vi "Periodic Tasks.vi"(8 "error in":errorcluster) -> ()   [LabVIEW 2017]
doc: "This VI runs in parallel to other tasks. It can contain as many user-defined periodic loops as you need. These can carry out PID or other sorts of timed response."
uses:
  <vilib>/Rock Robotics/WPI/Utilities/WPI_GetSetVariantRefNum.vi
  Robot Global Data.vi
  <vilib>/Rock Robotics/Network Tables/NT Write Numeric Array.vi
  <vilib>/Rock Robotics/Network Tables/NT Write Number.vi
  <vilib>/Rock Robotics/Network Tables/NT Write Boolean.vi
panel:
  out "ElevEnc":dbl
  out "LeftEncoder":dbl
  out "RightEncoder":dbl
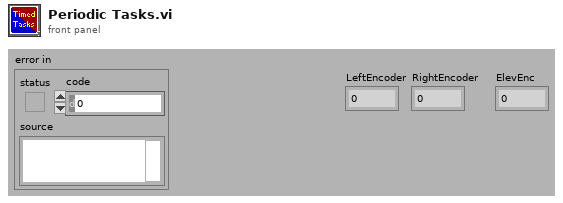
[diagram p1: front panel]
types:
  T1 = typedef "WPI_CompressorDevRef.ctl" = cluster{"DevStatus":errorcluster, "Pneumatics Control Module":u8}
  T2 = cluster{"Yaw":dbl, "Roll":dbl, "Pitch":dbl, "Heading":dbl, "Fused Heading":dbl}
  T3 = typedef "WPI_JoystickDevRef.ctl" = cluster{"Device":T4}
  T4 = typedef "WPI_JoystickDeviceEnum.ctl" = enum16{"USB 0", "USB 1", "USB 2", "USB 3", "USB 4", "USB 5"}
  T5 = typedef "WPI_DriverStationRobotMode2.ctl" = enum16{"Autonomous Disabled", "Autonomous Enabled", "Teleop Disabled", "Teleop Enabled", "Disconnected", "Finish", "Test Disabled", "Test Enabled", "Emergency Stopped"}
  T6 = cluster{"Buttons[0]":bool, "Buttons[1]":bool, "Buttons[2]":bool, "Buttons[3]":bool, "Buttons[4]":bool, "Buttons[5]":bool, "Buttons[6]":bool, "Buttons[7]":bool, "Buttons[8]":bool, "Buttons[9]":bool, "Buttons[10]":bool, "Buttons[11]":bool}
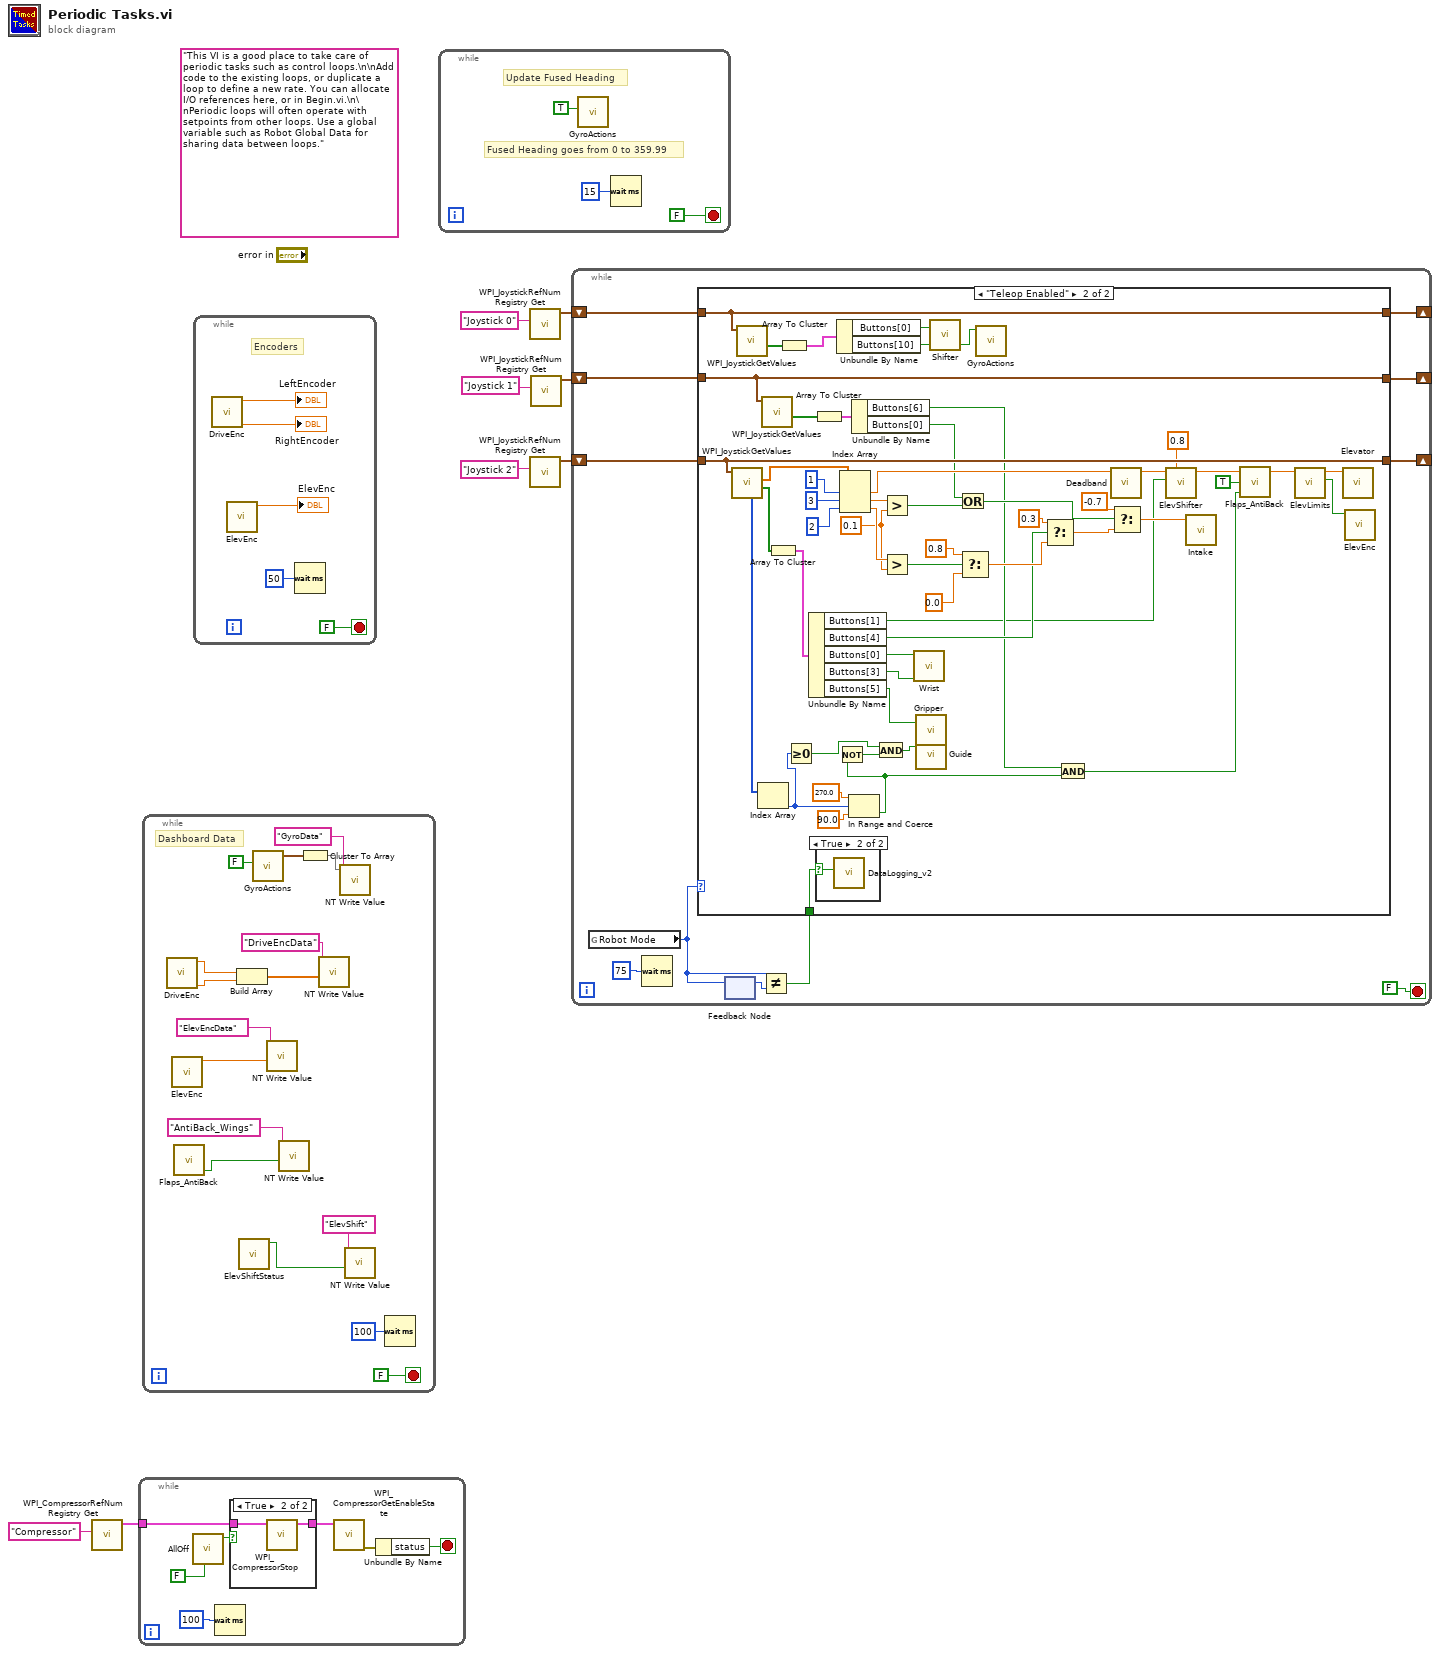
[diagram p0: block diagram]
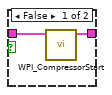
[diagram p4: hidden frame]
diagram:
  (unwired) "This VI is a good place to take care of periodic tasks such as control loops.\n\nAdd code to the existing loops, or duplicate a loop to define a new rate. You can allocate I/O references here, or in Begin.vi.\n\nPeriodic loops will often operate with setpoints from other loops. Use a global variable such as Robot Global Data for sharing data between loops."
  n1 = call <vilib>:"WPI_CompressorRefNum Registry Get.vi"("refnum name"="Compressor") -> ("CompressorDevRef"=w7:T1)  [unwired: 9 in, 1 out]
  n2 = while {
    tunnel: w7 -> [w13]
    stop <- w14 stop-if-true
    n3 = call "AllOff.vi"("Update?"=FALSE) -> ("Compressor"=w10:bool)  [unwired: 8 in, 2 out]
    n4 = Wait (ms)(milliseconds to wait=u32 100) -> ()  [unwired: 1 out]
    n5 = case shown="True" w10 {
      tunnel: w13 -> [w17 w19]
      tunnel: [w16 w18] -> w12
      frame False {
        n6 = call <vilib>:"WPI_CompressorStart.vi"("CompressorDevRef"=w17) -> ("CompressorDevRef"=w16:T1)  [unwired: 9 in, 1 out]
      }
      frame True {
        n7 = call <vilib>:"WPI_CompressorStop.vi"("CompressorDevRef"=w19) -> ("CompressorDevRef"=w18:T1)  [unwired: 9 in, 1 out]
      }
    }
    n8 = call <vilib>:"WPI_CompressorGetEnableState.vi"("CompressorDevRef"=w12) -> ("error out"=w11:errorcluster)  [unwired: 1 in, 9 out]
    n9 = Unbundle By Name(w11) -> ("status"=w14:bool)
  }
  n10 = while {
    stop <- FALSE stop-if-true
    # "Dashboard Data"
    n11 = call "DriveEnc.vi"() -> ("RightEncder"=w27:dbl, "LeftEncoder"=w28:dbl)  [unwired: 10 in]
    n12 = call "ElevEnc.vi"() -> ("ElevEnc"=w25:dbl)  [unwired: 11 in]
    n13 = call "Flaps_AntiBack.vi"() -> ("State"=w22:bool)  [unwired: 4 in, 1 out]
    n14 = Build Array(w28, w27) -> (w26:dbl[])
    n15 = call "ElevShiftStatus.vi"() -> ("ElevShiftStatusOut"=w20:bool)  [unwired: 11 in]
    n16 = call "GyroActions.vi"("Update?"=FALSE) -> ("YRPHfH"=w31:T2)  [unwired: 9 in, 1 out]
    n17 = call-poly <vilib>:"NT Write Value.vi"("Numeric"=w25, "Name"="ElevEncData") -> ()  [unwired: 9 in, 1 out]
    n18 = call-poly <vilib>:"NT Write Value.vi"("Boolean"=w22, "Name"="AntiBack_Wings") -> ()  [unwired: 9 in, 1 out]
    n19 = Cluster To Array(cluster=w31) -> (array=w35:dbl[])
    n20 = call-poly <vilib>:"NT Write Value.vi"("Numeric Array"=w26, "Name"="DriveEncData") -> ()  [unwired: 9 in, 1 out]
    n21 = call-poly <vilib>:"NT Write Value.vi"("Numeric Array"=w35, "Name"="GyroData") -> ()  [unwired: 9 in, 1 out]
    n22 = call-poly <vilib>:"NT Write Value.vi"("Boolean"=w20, "Name"="ElevShift") -> ()  [unwired: 9 in, 1 out]
    n23 = Wait (ms)(milliseconds to wait=u32 100) -> ()  [unwired: 1 out]
  }
  n24 = while {
    stop <- FALSE stop-if-true
    # "Encoders"
    n25 = call "DriveEnc.vi"() -> ("RightEncder"=→"RightEncoder":dbl, "LeftEncoder"=→"LeftEncoder":dbl)  [unwired: 10 in]
    n26 = call "ElevEnc.vi"() -> ("ElevEnc"=→"ElevEnc":dbl)  [unwired: 11 in]
    n27 = Wait (ms)(milliseconds to wait=u32 50) -> ()  [unwired: 1 out]
  }
  n28 = while {
    stop <- FALSE stop-if-true
    # "Update Fused Heading"
    # "Fused Heading goes from 0 to 359.99"
    n29 = call "GyroActions.vi"("Update?"=TRUE) -> ()  [unwired: 9 in, 2 out]
    n30 = Wait (ms)(milliseconds to wait=u32 15) -> ()  [unwired: 1 out]
  }
  n31 = call <vilib>:"WPI_JoystickRefNum Registry Get.vi"("refnum name"="Joystick 0") -> ("JoystickDevRef"=w5:T3)  [unwired: 9 in, 1 out]
  n32 = call <vilib>:"WPI_JoystickRefNum Registry Get.vi"("refnum name"="Joystick 2") -> ("JoystickDevRef"=w3:T3)  [unwired: 9 in, 1 out]
  n33 = call <vilib>:"WPI_JoystickRefNum Registry Get.vi"("refnum name"="Joystick 1") -> ("JoystickDevRef"=w1:T3)  [unwired: 9 in, 1 out]
  n34 = while {
    shift-right: [w52] -> _
    shift-left: w5 -> [w53]
    shift-right: [w49] -> _
    shift-left: w3 -> [w50]
    shift-right: [w47] -> _
    shift-left: w1 -> [w48]
    stop <- FALSE stop-if-true
    n35 = global read "Robot Global Data.vi" "Robot Mode"() -> (w45:T5)
    n36 = Wait (ms)(milliseconds to wait=u32 75) -> ()  [unwired: 1 out]
    n37 = feedback-in #1(w45) -> ()
    n38 = feedback #1() -> (w46:T5)  [unwired: 1 in]
    n39 = Not Equal?(x=w45, y=w46) -> (x != y?=w44:bool)
    n40 = case shown="\"Teleop Enabled\"" w45 {
      tunnel: w53 -> [w57 w109]
      tunnel: [w57 w109] -> w52
      tunnel: [w56 w106] -> w49
      tunnel: w50 -> [w56 w106]
      tunnel: [w55 w88] -> w47
      tunnel: w48 -> [w55 w88]
      tunnel: w44 -> [_ w75]
      frame "Teleop Disabled", Default {
      }
      frame "Teleop Enabled" {
        w91 = 0.1 ("y")
        n41 = call <vilib>:"WPI_JoystickGetValues.vi"("JoystickDevRef"=w106) -> ("Buttons"=w100:bool[], "Axes"=w82:dbl[], "POVs"=w73:i16[])  [unwired: 6 in, 2 out]
        n42 = call <vilib>:"WPI_JoystickGetValues.vi"("JoystickDevRef"=w109) -> ("Buttons"=w108:bool[])  [unwired: 6 in, 4 out]
        n43 = Index Array(array=w73) -> (element=w64:i16)  [unwired: 1 in]
        n44 = call <vilib>:"WPI_JoystickGetValues.vi"("JoystickDevRef"=w88) -> ("Buttons"=w89:bool[])  [unwired: 6 in, 4 out]
        n45 = Array To Cluster(array=w100) -> (cluster=w101:T6)
        n46 = Array To Cluster(array=w108) -> (cluster=w110:T6)
        n47 = Greater Or Equal To 0?(x=w64) -> (x >= 0?=w61:bool)
        n48 = Unbundle By Name(w101) -> ("Buttons[1]"=w58:bool, "Buttons[4]"=w84:bool, "Buttons[0]"=w87:bool, "Buttons[3]"=w86:bool, "Buttons[5]"=w83:bool)
        n49 = Array To Cluster(array=w89) -> (cluster=w90:T6)
        n50 = case shown="True" w75 {
          selector: w75 -> [_ w111]
          frame False {
          }
          frame True {
            n51 = call "DataLogging_v2.vi"("WriteToFile?"=w111) -> ()  [unwired: 9 in, 2 out]
          }
        }
        n52 = Unbundle By Name(w110) -> ("Buttons[0]"=w107:bool, "Buttons[10]"=w102:bool)
        n53 = Index Array(array=w82, index #1=1 ("index"), index #2=3 ("index"), index #3=2 ("index")) -> (element #1=w103:dbl, element #2=w93:dbl, element #3=w92:dbl)
        n54 = In Range and Coerce(upper limit=270.0, x=w64, lower limit=90.0) -> (In Range?=w65:bool)  [unwired: 1 out]
        n55 = Not(x=w65) -> (.not. x?=w63:bool)
        n56 = Unbundle By Name(w90) -> ("Buttons[6]"=w74:bool, "Buttons[0]"=w80:bool)
        n57 = And(x=w61, y=w63) -> (x .and. y?=w62:bool)
        n58 = Greater?(x=w93, y=w91) -> (0:w81:bool)
        n59 = Greater?(x=w92, y=w91) -> (0:w59:bool)
        n60 = call "Wrist.vi"("AllUp"=w86, "AllDown"=w87) -> ()  [unwired: 6 in]
        n61 = call "Gripper.vi"("Grip"=w83) -> ()  [unwired: 3 in]
        n62 = call "Guide.vi"("Shift?"=w62) -> ()  [unwired: 3 in]
        n63 = call "Shifter.vi"("Shift?"=w107) -> ()  [unwired: 3 in]
        n64 = Or(x=w80, y=w81) -> (x .or. y?=w79:bool)
        n65 = Select(t=0.8, s=w59, f=0.0) -> (s? t:f=w85:dbl)
        n66 = call "GyroActions.vi"("Zero"=w102) -> ()  [unwired: 9 in, 2 out]
        n67 = Select(t=0.3, s=w84, f=w85) -> (s? t:f=w98:dbl)
        n68 = And(x=w74, y=w65) -> (x .and. y?=w70:bool)
        n69 = call "Deadband.vi"("LeftPwrIn"=w103) -> ("LeftPwrOut"=w78:dbl)  [unwired: 9 in, 1 out]
        n70 = Select(t=-0.7, s=w79, f=w98) -> (s? t:f=w95:dbl)
        n71 = call "ElevShifter.vi"("MaxPwr"=0.8, "Shift?"=w58, "PwrIn"=w78) -> ("PwrOut"=w72:dbl)  [unwired: 6 in]
        n72 = call "Intake.vi"("Power"=w95) -> ()  [unwired: 11 in]
        n73 = call "Flaps_AntiBack.vi"("Toggle"=w70, "Update?"=TRUE, "MtrPwrIn"=w72) -> ("MtrPwrOut"=w71:dbl)  [unwired: 1 in, 1 out]
        n74 = call "ElevLimits.vi"("PowerIn"=w71) -> ("BotLimit"=w69:bool, "PowerOut"=w76:dbl)  [unwired: 8 in, 1 out]
        n75 = call "Elevator.vi"("Power"=w76) -> ()  [unwired: 11 in]
        n76 = call "ElevEnc.vi"("Reset?"=w69) -> ()  [unwired: 10 in, 1 out]
      }
    }
  }
